vi "Put Get.vi"(9 "Write Data":u8, 10 "Register Address":u8, 11 "Device Name":string="Basys2") -> (0 "Error Out":errorcluster, 2 "Read Data":u8)   [LabVIEW 2011, in "LVH-Adept.lvlib"]
uses:
  LVH-Adept.lvlib
  Private/DPCUTIL/DPCUTIL.lvlib
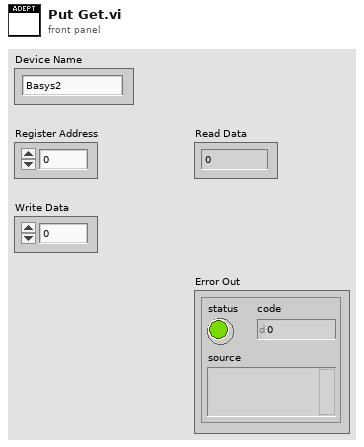
[diagram p1: front panel]
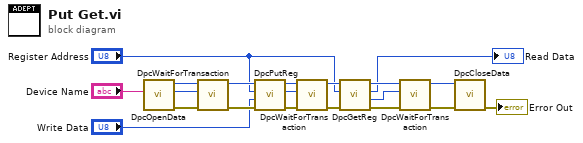
[diagram p0: block diagram]
diagram:
  n1 = call "DpcOpenData.vi"("Device Name"="Device Name") -> ("Error Out"=w20:errorcluster, "Task ID"=w6:u16, "Device Handle"=w10:u32)  [unwired: 8 in]
  n2 = call "DpcWaitForTransaction.vi"("Error In"=w20, "Task ID"=w6, "Device Handle"=w10) -> ("Error Out"=w17:errorcluster, "Device Handle"=w18:u32)  [unwired: 7 in]
  n3 = call "DpcPutReg.vi"("Error In"=w17, "Data"="Write Data", "Register Address"="Register Address", "Device Handle"=w18) -> ("Error Out"=w16:errorcluster, "Task ID"=w5:u16, "Device Hanle"=w15:u32)  [unwired: 5 in]
  n4 = call "DpcWaitForTransaction.vi"("Error In"=w16, "Task ID"=w5, "Device Handle"=w15) -> ("Error Out"=w9:errorcluster, "Device Handle"=w12:u32)  [unwired: 7 in]
  n5 = call "DpcGetReg.vi"("Error In"=w9, "Register Address"="Register Address", "Device Handle"=w12) -> ("Error Out"=w8:errorcluster, "Task ID"=w4:u16, "Data"=→"Read Data":u8, "Device Handle"=w7:u32)  [unwired: 5 in]
  n6 = call "DpcWaitForTransaction.vi"("Error In"=w8, "Task ID"=w4, "Device Handle"=w7) -> ("Error Out"=w13:errorcluster, "Device Handle"=w14:u32)  [unwired: 7 in]
  n7 = call "DpcCloseData.vi"("Error In"=w13, "Device Handle"=w14) -> ("Error Out"=→"Error Out":errorcluster)  [unwired: 8 in, 1 out]
